vi "Run.vi"(8 "error in (no error)":errorcluster caption="entrée d'erreur (pas d'erreur)", 10 "X":string[][](array[string]), 11 "minmax_scale.lvclass":refnum<class "minmax_scale.lvclass">) -> (0 "error out":errorcluster caption="sortie d'erreur", 2 "Data":T1, 3 "minmax_scale.lvclass":refnum<class "minmax_scale.lvclass">)   [LabVIEW 2020, in "minmax_scale.lvclass"]
uses:
  minmax_scale.lvclass
  minmax_scale.lvclass/minmax_scale.ctl
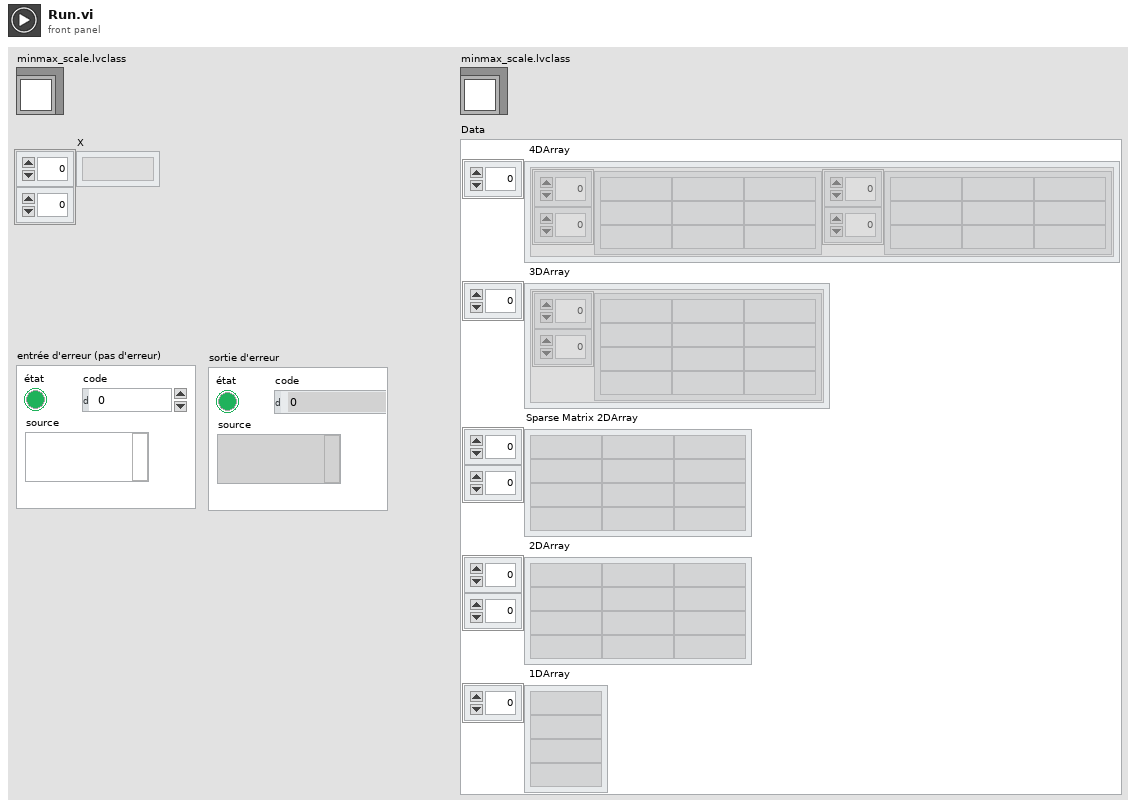
[diagram p1: front panel]
types:
  T1 = cluster{" 4DArray":cluster{"1":string[][], "2":string[][]}[], " 3DArray":cluster{"Tableau":string[][]}[], "Sparse Matrix 2DArray":string[][], " 2DArray":string[][], " 1DArray":string[]}
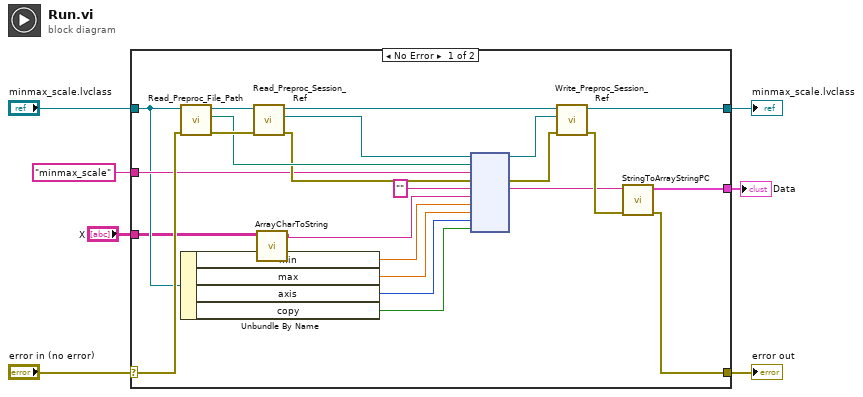
[diagram p0: block diagram]
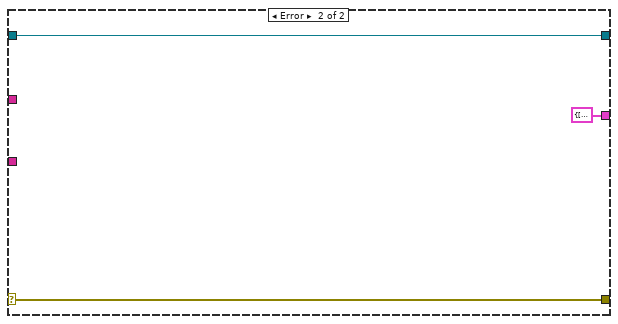
[diagram p2: hidden frame]
diagram:
  n1 = case shown="No Error" "error in (no error)" {
    selector: "error in (no error)" -> [w19 w33]
    tunnel: [w9 w33] -> w6
    tunnel: [w13 w32] -> w4
    tunnel: "minmax_scale.lvclass" -> [w17 w32]
    tunnel: "minmax_scale" ("Fonction") -> [w18 _]
    tunnel: [w10 T1 {" 4DArray"=[], " 3DArray"=[], "Sparse Matrix 2DArray"=[], " 2DArray"=[], " 1DArray"=[]} ("Data")] -> w1
    tunnel: "X" -> [w14 _]
    frame No Error {
      n2 = call-dynamic "Read_Preproc_File_Path.vi"("error in (no error)"=w19, "Python in"=w17) -> ("error out"=w29:errorcluster, "File_Path"=w26:path, "Python out"=w30:refnum<class "minmax_scale.lvclass">)  [unwired: 7 in]
      n3 = Unbundle By Name(w17) -> ("min"=w21:dbl, "max"=w20:dbl, "axis"=w16:i32, "copy"=w15:bool)
      n4 = call-dynamic "Read_Preproc_Session_Ref.vi"("error in (no error)"=w29, "Python in"=w30) -> ("error out"=w25:errorcluster, "Session_ref"=w27:refnum<k35>, "Python out"=w28:refnum<class "minmax_scale.lvclass">)  [unwired: 7 in]
      n5 = call "ArrayCharToString.vi"("TAB"=w14) -> ("Instruction"=w8:string)  [unwired: 10 in]
      n6 = node(w27, w26, w18, w25, "", w8, w21, w20, w16, w15) -> (w23:refnum<k35>, w24:errorcluster, w11:string)  [unwired: 5 in, 2 out]
      n7 = call-dynamic "Write_Preproc_Session_Ref.vi"("error in (no error)"=w24, "Session_ref"=w23, "Python in"=w28) -> ("error out"=w12:errorcluster, "Python out"=w13:refnum<class "minmax_scale.lvclass">)  [unwired: 7 in]
      n8 = call "StringToArrayStringPC.vi"("sortie d'erreur"=w12, "Return value"=w11) -> ("sortie d'erreur"=w9:errorcluster, "Data"=w10:T1)  [unwired: 8 in]
    }
    frame Error {
    }
  }
  "error out" <- w6
  "minmax_scale.lvclass" <- w4
  "Data" <- w1
